vi "Identify VIs Among Project Items.vi"(11 "Project Item References in":refnum<vi>[](array[refnum])) -> (2 "VI References":refnum<vi>[](array[refnum]), 3 "Project Item References out":refnum<vi>[](array[refnum]))   [LabVIEW 2020, in "Edit LVProj.lvlib"]
doc: "Given an array of project items, this subVI finds all the items that represent VIs and returns the VI references for those VIs."
uses:
  <vilib>/Utility/EditLVProj/Edit LVProj.lvlib
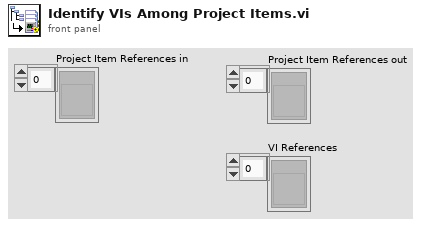
[diagram p1: front panel]
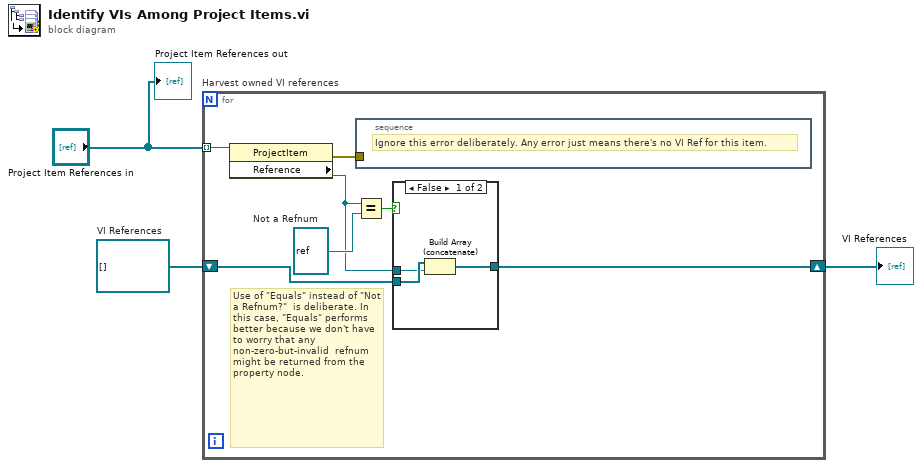
[diagram p0: block diagram]
diagram:
  w3 = refnum<vi>[] []  # VI References
  n1 = for "Harvest owned VI references" {
    tunnel: "Project Item References in" -> [w10] mode=indexing
    shift-right: [w6] -> w2
    shift-left: w3 -> [w7]
    w9 = refnum<vi> refnum  # Not a Refnum
    # "Use of \"Equals\" instead of \"Not a Refnum?\"  is deliberate. In this case, \"Equals\" performs better because we don't have to worry that any non-zero-but-invalid  refnum might be returned from the property node."
    n2 = property class="ProjectItem"(reference=w10) -> (error out=w4:errorcluster, "Reference"=w5:refnum<vi>)  [unwired: 1 in, 1 out]
    n3 = stacked-sequence {
      tunnel: w4 -> [_]
      frame #0 {
        # "Ignore this error deliberately. Any error just means there's no VI Ref for this item."
      }
    }
    n4 = Equal?(x=w5, y=w9) -> (x = y?=w8:bool)
    n5 = case shown="False" w8 {
      tunnel: w7 -> [w13 w14]
      tunnel: [w12 w14] -> w6
      tunnel: w5 -> [w11 _]
      frame False {
        n6 = Build Array (concatenate)(w13, w11) -> (w12:refnum<vi>[])
      }
      frame True {
      }
    }
  }
  "VI References" <- w2
  "Project Item References out" <- "Project Item References in"
